vi "Profiled PID Calculate.vi"(4 "Reset":bool, 5 "output saturation range":cluster{"output high":dbl, "output low":dbl}={"output high"=1.0, "output low"=-1.0}, 6 "PIDF gains":cluster{"Kp":dbl, "Ki":dbl, "Kd":dbl, "Kf":dbl}={"Kp"=5.0, "Ki"=0.0, "Kd"=0.0, "Kf"=0.0} {"Kf" format="%.3f"; "Kd" format="%.3f"; "Ki" format="%.3f"; "Kp" format="%.3f"}, 7 "Max Velocity":dbl=10.0 format="%#_13g", 8 "dt (s)":dbl, 9 "Output":dbl, 10 "setpoint":dbl(slide) scale=-100.0..100.0, 11 "Max Acceleration":dbl=10.0 format="%#_13g") -> (1 "output":dbl, 2 "Profiled Position":dbl, 3 "Profiled Velocity":dbl)   [LabVIEW 2019]
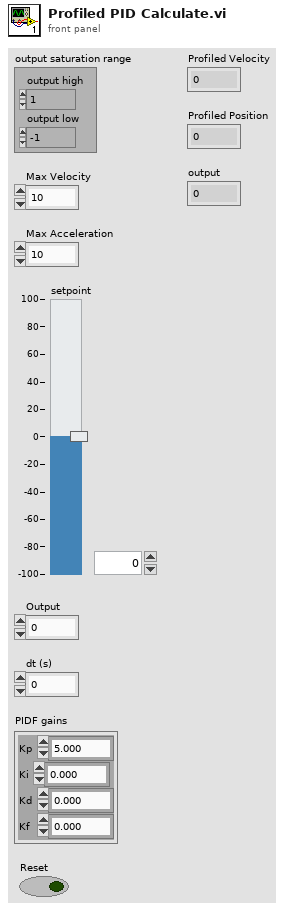
[diagram p1: front panel]
types:
  T1 = cluster{"PIDF Gains":cluster{"Kp":dbl, "Ki":dbl, "Kd":dbl, "Kf":dbl}, "Output Range":cluster{"output high":dbl, "output low":dbl}, "Profiled?":bool}
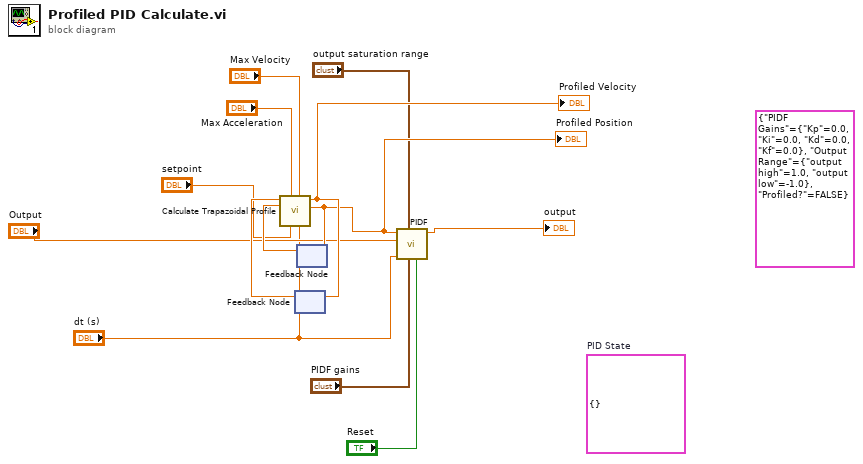
[diagram p0: block diagram]
diagram:
  (unwired) cluster{} {}  # PID State
  (unwired) T1 {"PIDF Gains"={"Kp"=0.0, "Ki"=0.0, "Kd"=0.0, "Kf"=0.0}, "Output Range"={"output high"=1.0, "output low"=-1.0}, "Profiled?"=FALSE}
  n1 = feedback #1() -> (w10:dbl)  [unwired: 1 in]
  n2 = feedback #2() -> (w9:dbl)  [unwired: 1 in]
  n3 = call "Calculate Trapazoidal Profile.vi"("t"="dt (s)", "Max Velocity"="Max Velocity", "Final Position"="setpoint", "Max Acceleration"="Max Acceleration", "Initial Position"=w9, "Initial Velocity"=w10) -> ("Result Position"=w11:dbl, "Result Velocity"=w12:dbl)  [unwired: 4 in]
  "Profiled Velocity" <- w12
  "Profiled Position" <- w11
  n4 = feedback-in #1(w12) -> ()
  n5 = feedback-in #2(w11) -> ()
  n6 = call "PIDF.vi"("reinitialize? (F)"="Reset", "PIDF gains"="PIDF gains", "output range"="output saturation range", "dt (s)"="dt (s)", "process variable"="Output", "setpoint"=w11) -> ("output"=→"output":dbl)  [unwired: 3 in, 2 out]
